vi "Messwert im Null-Bereich.vi"(8 "Toleranz Grundkalibrierung":sgl, 9 "Toleranz letzte KAL":sgl, 10 "Messwert":sgl, 11 "Rohwert":sgl) -> (0 "im Bereich":bool)   [LabVIEW 2020, in "ABB-EL3000.lvlib" / "Allgemeine VI.lvlib"]
uses:
  Allgemeine VI.lvlib
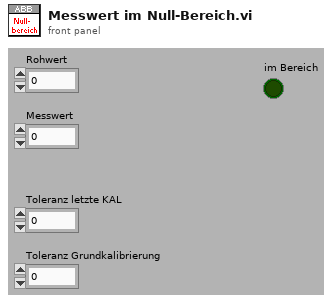
[diagram p1: front panel]
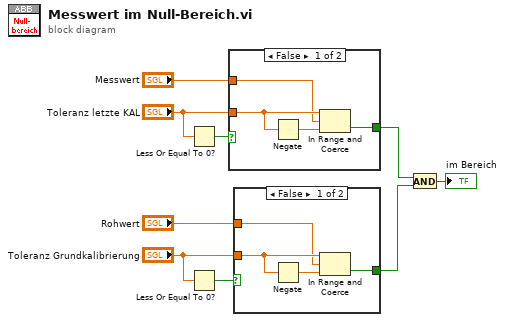
[diagram p0: block diagram]
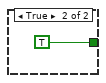
[diagram p2: hidden frame]
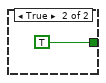
[diagram p3: hidden frame]
diagram:
  n1 = Less Or Equal To 0?(x="Toleranz letzte KAL") -> (x <= 0?=w5:bool)
  n2 = Less Or Equal To 0?(x="Toleranz Grundkalibrierung") -> (x <= 0?=w9:bool)
  n3 = case shown="False" w5 {
    tunnel: "Toleranz letzte KAL" -> [w12 _]
    tunnel: "Messwert" -> [w11 _]
    tunnel: [w10 TRUE] -> w3
    frame False {
      n4 = Negate(x=w12) -> (-x=w13:sgl)
      n5 = In Range and Coerce(upper limit=w12, x=w11, lower limit=w13) -> (In Range?=w10:bool)  [unwired: 1 out]
    }
    frame True {
    }
  }
  n6 = case shown="False" w9 {
    tunnel: "Toleranz Grundkalibrierung" -> [w17 _]
    tunnel: "Rohwert" -> [w16 _]
    tunnel: [w15 TRUE] -> w2
    frame False {
      n7 = Negate(x=w17) -> (-x=w18:sgl)
      n8 = In Range and Coerce(upper limit=w17, x=w16, lower limit=w18) -> (In Range?=w15:bool)  [unwired: 1 out]
    }
    frame True {
    }
  }
  n9 = And(x=w3, y=w2) -> (x .and. y?=→"im Bereich":bool)
